vi "content_type.vi"(11 "content_type":T1=enum."application/json") -> (3 "header":cluster{"header":string, "value":string}={"header"="Content-Type", "value"="application/json"})   [LabVIEW 2015, in "lv-dropbox.lvlib"]
uses:
  lv-dropbox.lvlib
  _controls/content_type.ctl
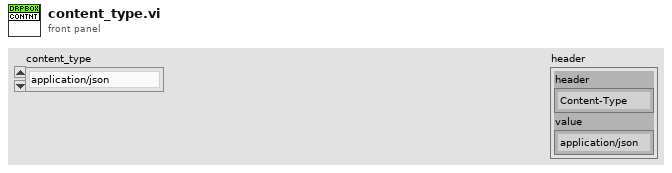
[diagram p1: front panel]
types:
  T1 = typedef "lv-dropbox.lvlib/content_type.ctl" = enum16{"<content_type>", "application/json", "application/octet-stream", "application/x-www-form-urlencoded"}
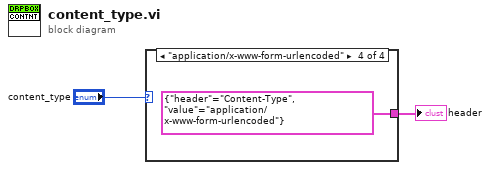
[diagram p0: block diagram]
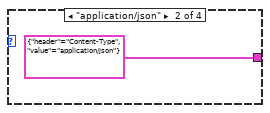
[diagram p3: hidden frame]
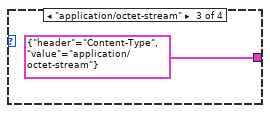
[diagram p4: hidden frame]
diagram:
  n1 = case shown="\"application/x-www-form-urlencoded\"" "content_type" {
    tunnel: [_ cluster{"header":string, "value":string} {"header"="Content-Type", "value"="application/json"} cluster{"header":string, "value":string} {"header"="Content-Type", "value"="application/octet-stream"} cluster{"header":string, "value":string} {"header"="Content-Type", "value"="application/x-www-form-urlencoded"}] -> w2
    frame Default {
    }
    frame "application/json" {
    }
    frame "application/octet-stream" {
    }
    frame "application/x-www-form-urlencoded" {
    }
  }
  "header" <- w2
